vi "Set Up TimeKeeper.vi"(8 "error in (no error)":errorcluster, 11 "RT Data Cluster in":T1={"Timekeeper hdl"="", "clkDisc session"=variant, "Compiled Data"={"SyncMod?"=FALSE, "SyncMod"="", "ConnectionSettings"={"Mode"=enum."Generate sample clock", "pxitrig"=FALSE, "pfi0"=FALSE, "pfi1"=FALSE, "pfi2"=FALSE, "External Pin"=enum."PFI0", "Routes"=[]}, "TimeKeeper"="", "ScanOffset(%)"=0.0, "StartDelay(s)"=0, "Time Ref Settings"={"Time Reference"=enum."GPS", "Priority 1"=0, "Priority 2"=0, "IRIG type"=enum."IRIGB AM", "Terminal"="", "PPSSetTime"=FALSE, "Start Time"=timestamp(0 s since 1904-01-01)}, "FIFO Locations"={"SysTime"=[], "TimeRef"=[], "Status"=[]}}, "OutputsData"=[], "OutputsFIFO"=refnum, "Scan Period"=0, "Timekeeper type"=enum."6683", "SyncMod type"=enum."6683", "SyncMod hdl"=""} {"Compiled Data"."Time Ref Settings"."Priority 2" min=0 max=255; "Compiled Data"."Time Ref Settings"."Priority 1" min=0 max=255}) -> (0 "error out":errorcluster, 3 "RT Data Cluster dup":T1={"Timekeeper hdl"="", "clkDisc session"=variant, "Compiled Data"={"SyncMod?"=FALSE, "SyncMod"="", "ConnectionSettings"={"Mode"=enum."Generate sample clock", "pxitrig"=FALSE, "pfi0"=FALSE, "pfi1"=FALSE, "pfi2"=FALSE, "External Pin"=enum."PFI0", "Routes"=[]}, "TimeKeeper"="", "ScanOffset(%)"=0.0, "StartDelay(s)"=0, "Time Ref Settings"={"Time Reference"=enum."GPS", "Priority 1"=0, "Priority 2"=0, "IRIG type"=enum."IRIGB AM", "Terminal"="", "PPSSetTime"=FALSE, "Start Time"=timestamp(0 s since 1904-01-01)}, "FIFO Locations"={"SysTime"=[], "TimeRef"=[], "Status"=[]}}, "OutputsData"=[], "OutputsFIFO"=refnum, "Scan Period"=0, "Timekeeper type"=enum."6683", "SyncMod type"=enum."6683", "SyncMod hdl"=""} {"Compiled Data"."Time Ref Settings"."Priority 2" min=0 max=255; "Compiled Data"."Time Ref Settings"."Priority 1" min=0 max=255})   [LabVIEW 2017, in "Chassis TimeSync Engine.lvlib"]
uses:
  Chassis TimeSync Engine.lvlib
  RT Data Cluster.ctl
  mdevClkDisc.llb/_clkDisc_session.ctl
  Shared/Compiled Data.ctl
  Shared/Connection Settings.ctl
  Shared/Mode.ctl
  Shared/External Pin.ctl
  Shared/Routes.ctl
  Shared/Route.ctl
  Shared/Time Ref Settings.ctl
  Shared/Time Reference.ctl
  Shared/IRIG Type.ctl
  timekeeper type.ctl
  <instrlib>/niSync/niSync.llb/niSync Set Time Reference (GPS).vi
  <instrlib>/niSync/niSync.llb/niSync Set Time Reference (Free Running).vi
  <instrlib>/niSync/niSync.llb/niSync Set Time Reference (1588 Ordinary Clock).vi
  <instrlib>/niSync/niSync.llb/niSync Set Time Reference (PPS).vi
  <instrlib>/niSync/niSync.llb/niSync Set Time Reference (IRIG).vi
  Shared/Chassis TimeSync Shared.lvlib
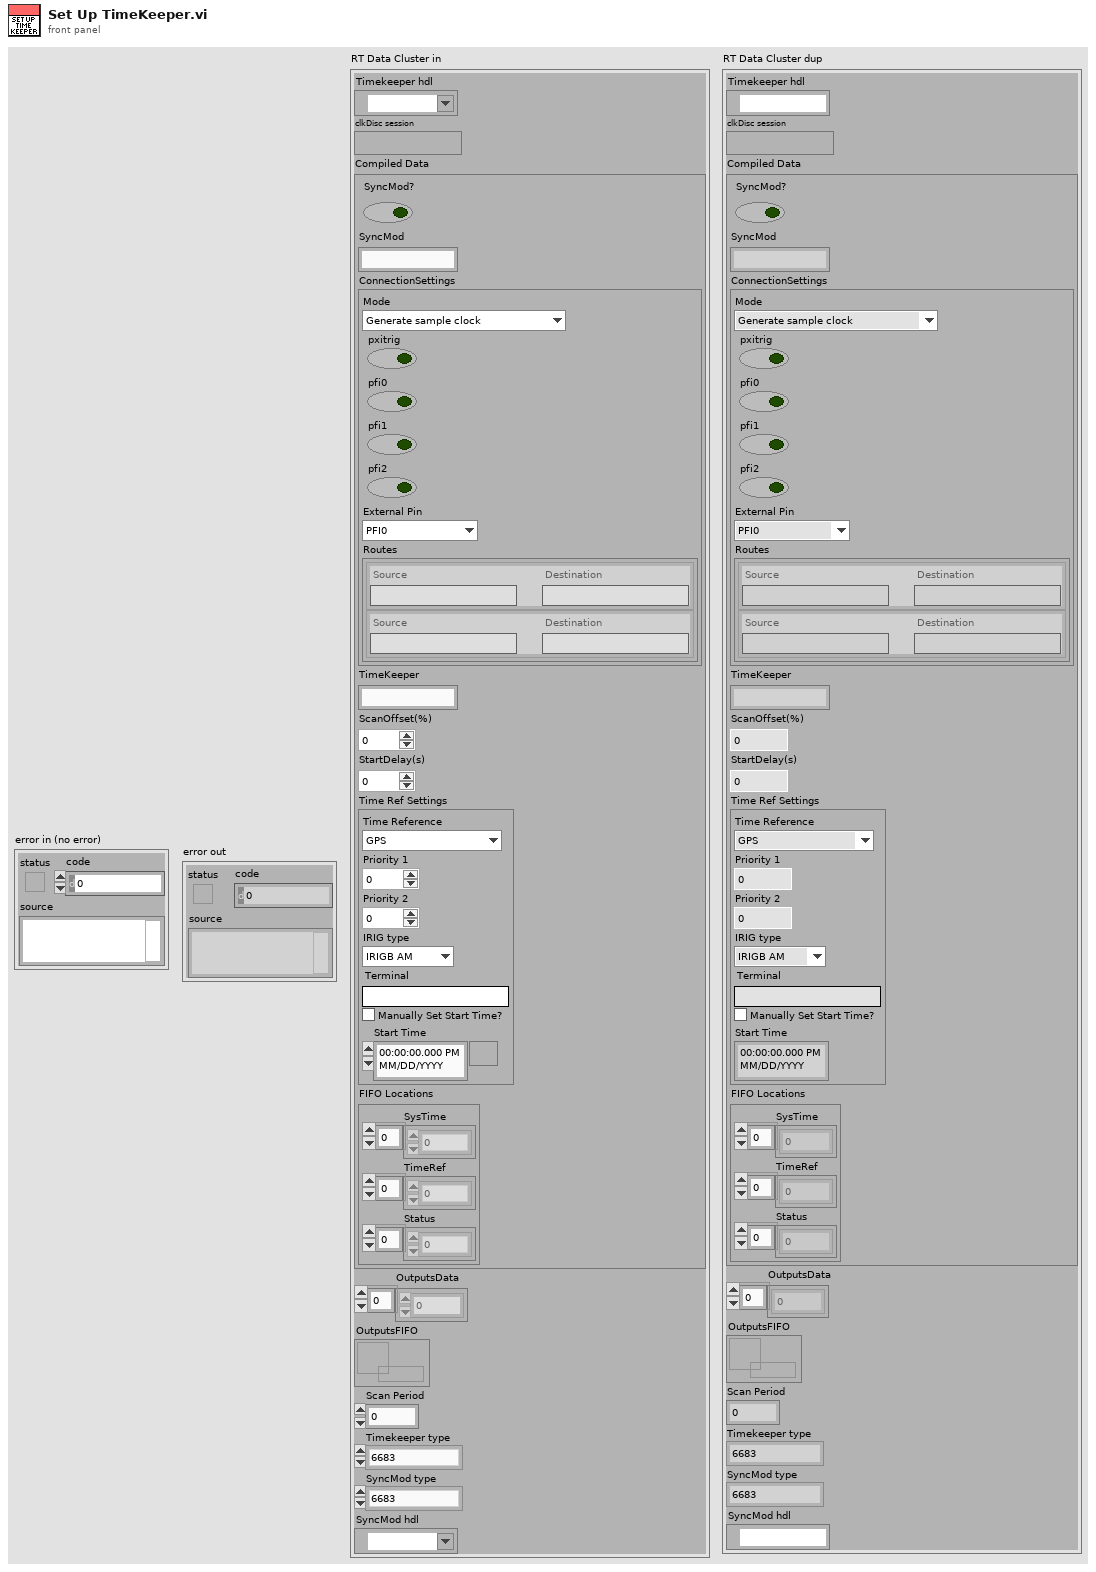
[diagram p1: front panel]
types:
  T1 = typedef "Chassis TimeSync Engine.lvlib/RT Data Cluster.ctl" = cluster{"Timekeeper hdl":refnum<k15>, "clkDisc session":T2, "Compiled Data":T3, "OutputsData":dbl[], "OutputsFIFO":refnum<k33>, "Scan Period":u32, "Timekeeper type":T12, "SyncMod type":T12, "SyncMod hdl":refnum<k15>}
  T2 = typedef "_clkDisc_session.ctl" = variant
  T3 = typedef "Chassis TimeSync Shared.lvlib/Compiled Data.ctl" = cluster{"SyncMod?":bool, "SyncMod":string, "ConnectionSettings":T4, "TimeKeeper":string, "ScanOffset(%)":dbl, "StartDelay(s)":u16, "Time Ref Settings":T9, "FIFO Locations":cluster{"SysTime":i32[], "TimeRef":i32[], "Status":i32[]}}
  T4 = typedef "Chassis TimeSync Shared.lvlib/Connection Settings.ctl" = cluster{"Mode":T5, "pxitrig":bool, "pfi0":bool, "pfi1":bool, "pfi2":bool, "External Pin":T6, "Routes":T7}
  T5 = typedef "Chassis TimeSync Shared.lvlib/Mode.ctl" = enum16{"Generate sample clock", "Route sample clock out of chassis", "Route sample clock into chassis", "Custom routes"}
  T6 = typedef "Chassis TimeSync Shared.lvlib/External Pin.ctl" = enum16{"PFI0", "PFI1", "PFI2"}
  T7 = typedef "Chassis TimeSync Shared.lvlib/Routes.ctl" = T8[]
  T8 = typedef "Chassis TimeSync Shared.lvlib/Route.ctl" = cluster{"Source":string, "Destination":string}
  T9 = typedef "Chassis TimeSync Shared.lvlib/Time Ref Settings.ctl" = cluster{"Time Reference":T10, "Priority 1":i32, "Priority 2":i32, "IRIG type":T11, "Terminal":string, "PPSSetTime":bool, "Start Time":timestamp}
  T10 = typedef "Chassis TimeSync Shared.lvlib/Time Reference.ctl" = enum16{"GPS", "IRIG", "PPS", "1588 Ordinary Clock", "PXI Chassis Clock", "Free Running (Internal)"}
  T11 = typedef "Chassis TimeSync Shared.lvlib/IRIG Type.ctl" = enum16{"IRIGB DC", "IRIGB AM"}
  T12 = typedef "Chassis TimeSync Engine.lvlib/timekeeper type.ctl" = enum16{"6683", "6683H", "6682", "6682H", "non-timekeeper", "timekeeper"}
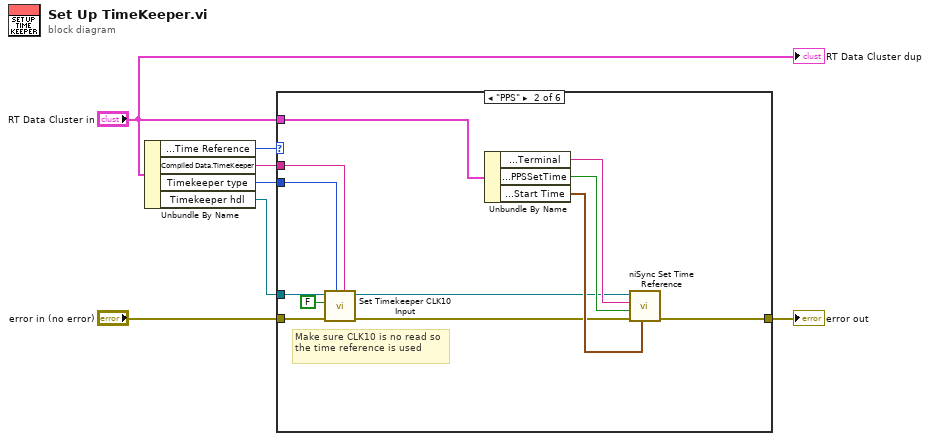
[diagram p0: block diagram]
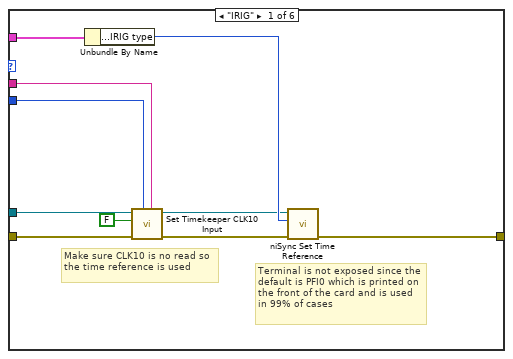
[diagram p2: hidden frame]
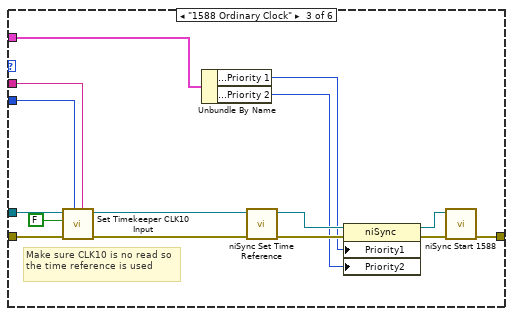
[diagram p3: hidden frame]
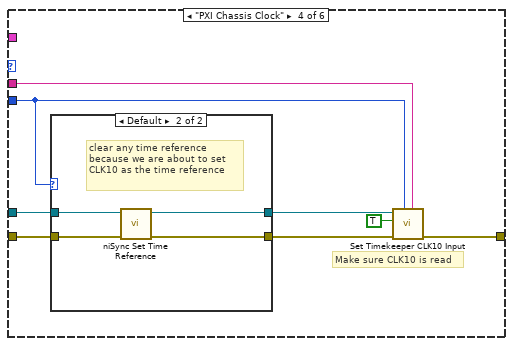
[diagram p4: hidden frame]
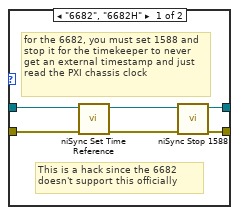
[diagram p5: hidden frame]
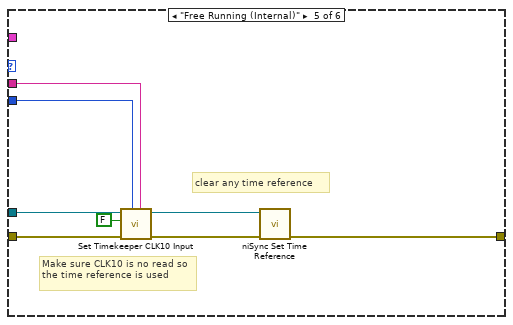
[diagram p6: hidden frame]
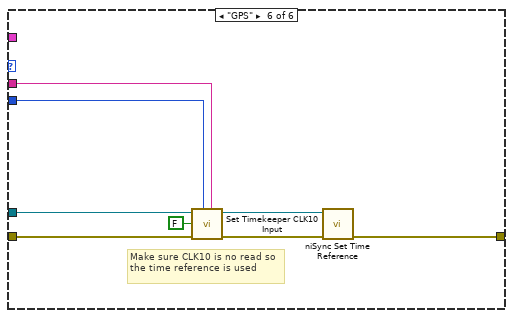
[diagram p7: hidden frame]
diagram:
  n1 = Unbundle By Name("RT Data Cluster in") -> ("Compiled Data.Time Ref Settings.Time Reference"=w6:T10, "Compiled Data.TimeKeeper"=w1:string, "Timekeeper type"=w2:T12, "Timekeeper hdl"=w5:refnum<k15>)
  n2 = case shown="\"PPS\"" w6 {
    tunnel: "error in (no error)" -> [w11 w29 w33 w51 w70 w74]
    tunnel: w5 -> [w12 w22 w35 w52 w67 w75]
    tunnel: "RT Data Cluster in" -> [w17 w28 w44 _ _ _]
    tunnel: [w15 w26 w37 w50 w69 w78] -> w3
    tunnel: w2 -> [w9 w20 w31 w45 w65 w72]
    tunnel: w1 -> [w8 w18 w30 w49 w64 w71]
    frame "IRIG" {
      # "Make sure CLK10 is no read so the time reference is used"
      # "Terminal is not exposed since the default is PFI0 which is printed on the front of the card and is used in 99% of cases"
      n3 = Unbundle By Name(w17) -> ("Compiled Data.Time Ref Settings.IRIG type"=w16:T11)
      n4 = call "Set Timekeeper CLK10 Input.vi"("Timekeeper"=w8, "Timekeeper type"=w9, "error in (no error)"=w11, "Enabled?"=FALSE ("Advanced:Time Reference:Clk10 Disciplining Enabled"), "timekeeper in"=w12) -> ("error out"=w14:errorcluster, "timekeeper out"=w13:refnum<k15>)  [unwired: 5 in]
      n5 = call-poly <instrlib>:"niSync Set Time Reference.vi"("error in (no error)"=w14, "IRIG type"=w16, "instrument handle"=w13) -> ("error out"=w15:errorcluster)  [unwired: 7 in, 1 out]
    }
    frame "PPS" {
      # "Make sure CLK10 is no read so the time reference is used"
      n6 = call "Set Timekeeper CLK10 Input.vi"("Timekeeper"=w18, "Timekeeper type"=w20, "error in (no error)"=w29, "Enabled?"=FALSE, "timekeeper in"=w22) -> ("error out"=w23:errorcluster, "timekeeper out"=w21:refnum<k15>)  [unwired: 5 in]
      n7 = Unbundle By Name(w28) -> ("Compiled Data.Time Ref Settings.Terminal"=w27:string, "Compiled Data.Time Ref Settings.PPSSetTime"=w25:bool, "Compiled Data.Time Ref Settings.Start Time"=w24:timestamp)
      n8 = call-poly <instrlib>:"niSync Set Time Reference.vi"("initial time"=w24, "error in (no error)"=w23, "use manual time"=w25, "terminal"=w27, "instrument handle"=w21) -> ("error out"=w26:errorcluster)  [unwired: 5 in, 1 out]
    }
    frame "1588 Ordinary Clock" {
      # "Make sure CLK10 is no read so the time reference is used"
      n9 = call "Set Timekeeper CLK10 Input.vi"("Timekeeper"=w30, "Timekeeper type"=w31, "error in (no error)"=w33, "Enabled?"=FALSE ("Advanced:Time Reference:Clk10 Disciplining Enabled"), "timekeeper in"=w35) -> ("error out"=w36:errorcluster, "timekeeper out"=w34:refnum<k15>)  [unwired: 5 in]
      n10 = Unbundle By Name(w44) -> ("Compiled Data.Time Ref Settings.Priority 1"=w41:i32, "Compiled Data.Time Ref Settings.Priority 2"=w40:i32)
      n11 = call-poly <instrlib>:"niSync Set Time Reference.vi"("error in (no error)"=w36, "instrument handle"=w34) -> ("error out"=w43:errorcluster, "instrument handle out"=w42:refnum<k15>)  [unwired: 8 in]
      n12 = property class="niSync"(reference=w42, error in=w43, "Priority1"=w41, "Priority2"=w40) -> (reference out=w38:refnum<k15>, error out=w39:errorcluster)
      n13 = call <instrlib>:"niSync Start 1588.vi"("error in (no error)"=w39, "instrument handle"=w38) -> ("error out"=w37:errorcluster)  [unwired: 8 in, 1 out]
    }
    frame "PXI Chassis Clock" {
      # "Make sure CLK10 is read"
      n14 = case shown="Default" w45 {
        tunnel: w52 -> [w58 w62]
        tunnel: w51 -> [w57 w61]
        tunnel: [w54 w59] -> w48
        tunnel: [w53 w60] -> w47
        frame "6682", "6682H" {
          # "This is a hack since the 6682 doesn't support this officially"
          # "for the 6682, you must set 1588 and stop it for the timekeeper to never get an external timestamp and just read the PXI chassis clock"
          n15 = call-poly <instrlib>:"niSync Set Time Reference.vi"("error in (no error)"=w57, "instrument handle"=w58) -> ("error out"=w56:errorcluster, "instrument handle out"=w55:refnum<k15>)  [unwired: 8 in]
          n16 = call <instrlib>:"niSync Stop 1588.vi"("error in (no error)"=w56, "instrument handle"=w55) -> ("error out"=w53:errorcluster, "instrument handle out"=w54:refnum<k15>)  [unwired: 8 in]
        }
        frame Default {
          # "clear any time reference because we are about to set CLK10 as the time reference"
          n17 = call-poly <instrlib>:"niSync Set Time Reference.vi"("error in (no error)"=w61, "instrument handle"=w62) -> ("error out"=w60:errorcluster, "instrument handle out"=w59:refnum<k15>)  [unwired: 8 in]
        }
      }
      n18 = call "Set Timekeeper CLK10 Input.vi"("Timekeeper"=w49, "Timekeeper type"=w45, "error in (no error)"=w47, "Enabled?"=TRUE ("Advanced:Time Reference:Clk10 Disciplining Enabled"), "timekeeper in"=w48) -> ("error out"=w50:errorcluster)  [unwired: 5 in, 1 out]
    }
    frame "Free Running (Internal)" {
      # "Make sure CLK10 is no read so the time reference is used"
      # "clear any time reference"
      n19 = call "Set Timekeeper CLK10 Input.vi"("Timekeeper"=w64, "Timekeeper type"=w65, "error in (no error)"=w70, "Enabled?"=FALSE, "timekeeper in"=w67) -> ("error out"=w68:errorcluster, "timekeeper out"=w66:refnum<k15>)  [unwired: 5 in]
      n20 = call-poly <instrlib>:"niSync Set Time Reference.vi"("error in (no error)"=w68, "instrument handle"=w66) -> ("error out"=w69:errorcluster)  [unwired: 8 in, 1 out]
    }
    frame "GPS" {
      # "Make sure CLK10 is no read so the time reference is used"
      n21 = call "Set Timekeeper CLK10 Input.vi"("Timekeeper"=w71, "Timekeeper type"=w72, "error in (no error)"=w74, "Enabled?"=FALSE ("Advanced:Time Reference:Clk10 Disciplining Enabled"), "timekeeper in"=w75) -> ("error out"=w77:errorcluster, "timekeeper out"=w76:refnum<k15>)  [unwired: 5 in]
      n22 = call-poly <instrlib>:"niSync Set Time Reference.vi"("error in (no error)"=w77, "instrument handle"=w76) -> ("error out"=w78:errorcluster)  [unwired: 8 in, 1 out]
    }
  }
  "error out" <- w3
  "RT Data Cluster dup" <- "RT Data Cluster in"
